vi "Size UI.vi"(0 "VI":refnum<vi>, 1 "Decoration":refnum<vi>, 5 "Line Numbers":refnum<vi>, 7 "Scrollbar":refnum<vi>, 9 "Strings":refnum<vi>[](array[refnum]), 11 "error in (no error)":errorcluster) -> (15 "error out":errorcluster)   [LabVIEW 2016, in "Code String LV.lvclass"]
doc: "Performs the logic to appropriately size and align all the UI components.\n--------------------\nCopyright (c) 2019 Analog Devices, Inc. All rights reserved.\n\nRedistribution and use in source and binary forms, with or without modification,\nare permitted provided that the following conditions are met:\n - Redistributions of source code must retain the above copyright notice, this\n list of conditions and the following disclaimer.\n - Redistributions in binary form must reproduce the above copyright notice,\n this list of conditions and the following disclaimer in the documentation\n and/or other materials provided with the distribution.\n - Modified versions of the software must be conspicuously marked as such.\n - This software is licensed solely and exclusively for use with\n processors/products manufactured by or for Analog Devices, Inc.\n - This software may not be combined or merged with other code in any manner\n that would cause the software to become subject to terms and conditions\n which differ from those listed here.\n - Neither the name of Analog Devices, Inc. nor the names of its contributors\n may be used to endorse or promote products derived from this software\n without specific prior written permission.\n - The use of this software may or may not infringe the patent rights of one or\n more patent holders. This license does not release you from the requirement\n that you obtain separate licenses from these patent holders to use this\n software.\n\nTHIS SOFTWARE IS PROVIDED BY ANALOG DEVICES, INC. AND CONTRIBUTORS \"AS IS\" AND\nANY EXPRESS OR IMPLIED WARRANTIES, INCLUDING, BUT NOT LIMITED TO,\nNON-INFRINGEMENT, TITLE, MERCHANTABILITY AND FITNESS FOR A PARTICULAR PURPOSE\nARE DISCLAIMED. IN NO EVENT SHALL ANALOG DEVICES, INC. OR CONTRIBUTORS BE LIABLE\nFOR ANY DIRECT, INDIRECT, INCIDENTAL, SPECIAL, EXEMPLARY, PUNITIVE OR\nCONSEQUENTIAL DAMAGES (INCLUDING, BUT NOT LIMITED TO, DAMAGES ARISING OUT OF\nCLAIMS OF INTELLECTUAL PROPERTY RIGHTS INFRINGEMENT; PROCUREMENT OF SUBSTITUTE\nGOODS OR SERVICES; LOSS OF USE, DATA, OR PROFITS; OR BUSINESS INTERRUPTION)\nHOWEVER CAUSED AND ON ANY THEORY OF LIABILITY, WHETHER IN CONTRACT, STRICT\nLIABILITY, OR TORT (INCLUDING NEGLIGENCE OR OTHERWISE) ARISING IN ANY WAY OUT OF\nTHE USE OF THIS SOFTWARE, EVEN IF ADVISED OF THE POSSIBILITY OF SUCH DAMAGE.\n\n2019-01-10-7CBSD SLA"
uses:
  Code String LV.lvclass
panel:
  # "Copyright (c) 2019 Analog Devices, Inc.  All rights reserved.\n\nRedistribution and use in source and binary forms, with or without modification,\nare permitted provided that the following conditions are met:\n  - Redistributions of source code must retain the above copyright notice, this\n    list of conditions and the following disclaimer.\n  - Redistributions in binary form must reproduce the above copyright notice,\n    this list of conditions and the following disclaimer in the documentation\n    and/or other materials provided with the distribution.\n  - Modified versions of the software must be conspicuously marked as such.\n  - This software is licensed solely and exclusively for use with\n    processors/products manufactured by or for Analog Devices, Inc.\n  - This software may not be combined or merged with other code in any manner\n    that would cause the software to become subject to terms and conditions\n    which differ from those listed here.\n  - Neither the name of Analog Devices, Inc. nor the names of its contributors\n    may be used to endorse or promote products derived from this software\n    without specific prior written permission.\n  - The use of this software may or may not infringe the patent rights of one or\n    more patent holders.  This license does not release you from the requirement\n    that you obtain separate licenses from these patent holders to use this\n    software.\n\nTHIS SOFTWARE IS PROVIDED BY ANALOG DEVICES, INC. AND CONTRIBUTORS \"AS IS\" AND\nANY EXPRESS OR IMPLIED WARRANTIES, INCLUDING, BUT NOT LIMITED TO,\nNON-INFRINGEMENT, TITLE, MERCHANTABILITY AND FITNESS FOR A PARTICULAR PURPOSE\nARE DISCLAIMED. IN NO EVENT SHALL ANALOG DEVICES, INC. OR CONTRIBUTORS BE LIABLE\nFOR ANY DIRECT, INDIRECT, INCIDENTAL, SPECIAL, EXEMPLARY, PUNITIVE OR\nCONSEQUENTIAL DAMAGES (INCLUDING, BUT NOT LIMITED TO, DAMAGES ARISING OUT OF\nCLAIMS OF INTELLECTUAL PROPERTY RIGHTS INFRINGEMENT; PROCUREMENT OF SUBSTITUTE\nGOODS OR SERVICES; LOSS OF USE, DATA, OR PROFITS; OR BUSINESS INTERRUPTION)\nHOWEVER CAUSED AND ON ANY THEORY OF LIABILITY, WHETHER IN CONTRACT, STRICT\nLIABILITY, OR TORT (INCLUDING NEGLIGENCE OR OTHERWISE) ARISING IN ANY WAY OUT OF\nTHE USE OF THIS SOFTWARE, EVEN IF ADVISED OF THE POSSIBILITY OF SUCH DAMAGE.\n\n2019-01-10-7CBSD SLA"
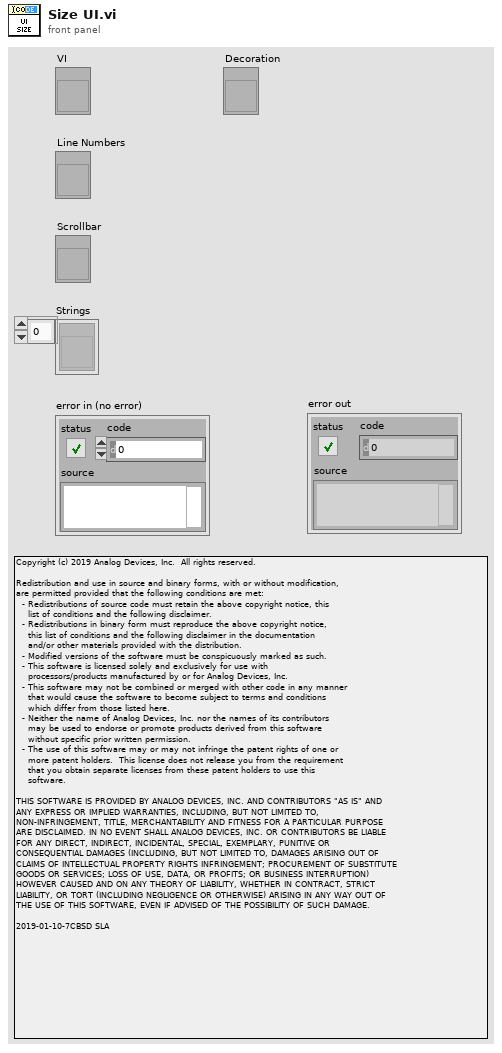
[diagram p1: front panel]
types:
  T1 = typedef "LVBoundsTypeDef.ctl" = cluster{"Width":u32, "Height":u32}
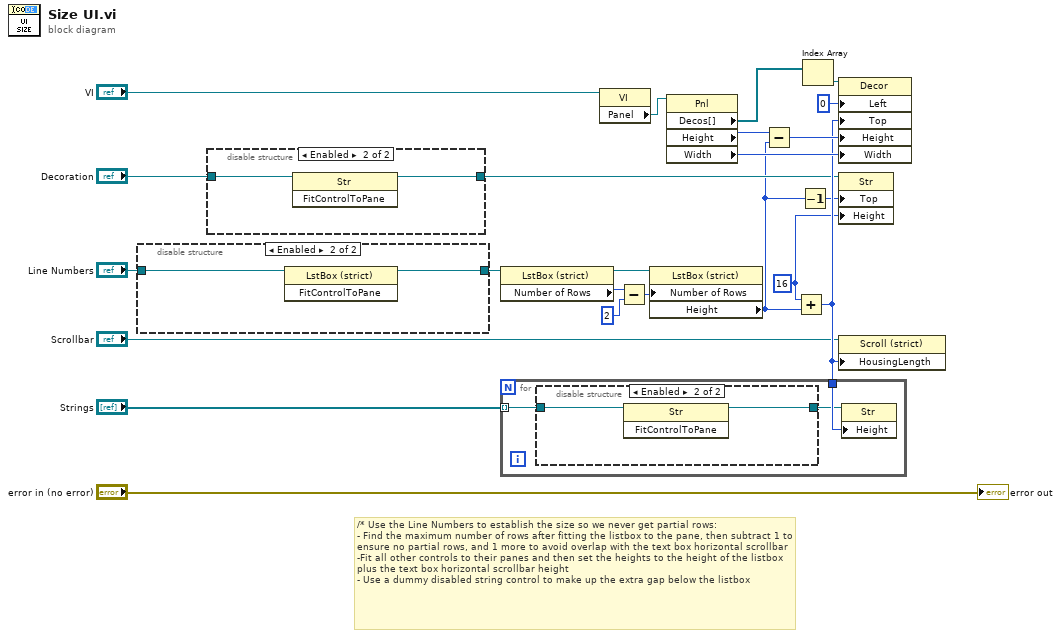
[diagram p0: block diagram]
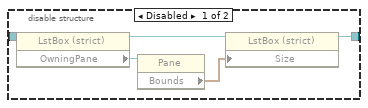
[diagram p2: hidden frame]
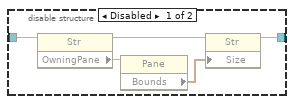
[diagram p3: hidden frame]
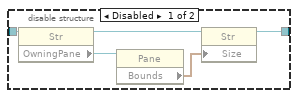
[diagram p4: hidden frame]
diagram:
  w2 = u32 16 ("x")
  # "/* Use the Line Numbers to establish the size so we never get partial rows:\n- Find the maximum number of rows after fitting the listbox to the pane, then subtract 1 to ensure no partial rows, and 1 more to avoid overlap with the text box horizontal scrollbar\n-Fit all other controls to their panes and then set the heights to the height of the listbox plus the text box horizontal scrollbar height\n- Use a dummy disabled string control to make up the extra gap below the listbox"
  n1 = disable-structure shown="Enabled" {
    disable-tunnel: "Line Numbers" -> [w28 w30]
    disable-tunnel: [w24 w29] -> w5
    frame Disabled {
      n2 = property class="LstBox (strict)"(reference=w28) -> (reference out=w25:refnum<vi>, "OwningPane"=w26:refnum<vi>)  [unwired: 1 in, 1 out]
      n3 = property class="Pane"(reference=w26) -> ("Bounds"=w27:T1)  [unwired: 1 in, 2 out]
      n4 = property class="LstBox (strict)"(reference=w25, "Size"=w27) -> (reference out=w24:refnum<vi>)  [unwired: 1 in, 1 out]
    }
    frame Enabled {
      n5 = invoke class="LstBox (strict)" method="FitControlToPane"(reference=w30) -> (reference out=w29:refnum<vi>)  [unwired: 2 in, 2 out]
    }
  }
  n6 = disable-structure shown="Enabled" {
    disable-tunnel: "Decoration" -> [w35 w37]
    disable-tunnel: [w32 w36] -> w6
    frame Disabled {
      n7 = property class="Str"(reference=w35) -> (reference out=w34:refnum<vi>, "OwningPane"=w33:refnum<vi>)  [unwired: 1 in, 1 out]
      n8 = property class="Pane"(reference=w33) -> ("Bounds"=w31:T1)  [unwired: 1 in, 2 out]
      n9 = property class="Str"(reference=w34, "Size"=w31) -> (reference out=w32:refnum<vi>)  [unwired: 1 in, 1 out]
    }
    frame Enabled {
      n10 = invoke class="Str" method="FitControlToPane"(reference=w37) -> (reference out=w36:refnum<vi>)  [unwired: 2 in, 2 out]
    }
  }
  n11 = property on="Property Node" class="LstBox (strict)"(reference=w5) -> (reference out=w8:refnum<vi>, "Number of Rows"=w7:u32)  [unwired: 1 in, 1 out]
  n12 = property on="Property Node" class="VI"(reference="VI") -> ("Panel"=w21:refnum<vi>)  [unwired: 1 in, 2 out]
  n13 = Subtract(x=w7, y=u32 2 ("x")) -> (x-y=w10:u32)
  n14 = property on="Property Node" class="LstBox (strict)"(reference=w8, "Number of Rows"=w10) -> ("Height"=w3:u32)  [unwired: 1 in, 2 out]
  n15 = property on="Property Node" class="Pnl"(reference=w21) -> ("Decos[]"=w20:refnum<vi>[], "Height"=w22:u32, "Width"=w23:u32)  [unwired: 1 in, 2 out]
  n16 = Subtract(x=w22, y=w3) -> (x-y=w14:u32)
  n17 = Add(x=w2, y=w3) -> (x+y=w13:u32)
  n18 = for {
    tunnel: "Strings" -> [w39] mode=indexing
    tunnel: w13 -> [w40]
    n19 = disable-structure shown="Enabled" {
      disable-tunnel: w39 -> [w42 w47]
      disable-tunnel: [w41 w46] -> w38
      frame Disabled {
        n20 = property class="Str"(reference=w42) -> (reference out=w43:refnum<vi>, "OwningPane"=w44:refnum<vi>)  [unwired: 1 in, 1 out]
        n21 = property class="Pane"(reference=w44) -> ("Bounds"=w45:T1)  [unwired: 1 in, 2 out]
        n22 = property class="Str"(reference=w43, "Size"=w45) -> (reference out=w41:refnum<vi>)  [unwired: 1 in, 1 out]
      }
      frame Enabled {
        n23 = invoke class="Str" method="FitControlToPane"(reference=w47) -> (reference out=w46:refnum<vi>)  [unwired: 2 in, 2 out]
      }
    }
    n24 = property class="Str"(reference=w38, "Height"=w40) -> ()  [unwired: 1 in, 2 out]
  }
  n25 = Decrement(x=w3) -> (x-1=w1:u32)
  n26 = Index Array(array=w20) -> (element=w11:refnum<vi>)  [unwired: 1 in]
  n27 = property on="Property Node" class="Decor"(reference=w11, "Left"=0 ("Position:Left"), "Top"=w13, "Height"=w14, "Width"=w23) -> ()  [unwired: 1 in, 2 out]
  n28 = property on="Property Node" class="Str"(reference=w6, "Top"=w1, "Height"=w2) -> ()  [unwired: 1 in, 2 out]
  n29 = property on="Property Node" class="Scroll (strict)"(reference="Scrollbar", "HousingLength"=w13) -> ()  [unwired: 1 in, 2 out]
  "error out" <- "error in (no error)"
